vi "Wall Correction.vi"(8 "Direction from car (rad)":dbl[](array[numeric]), 9 "Distance form car":dbl[](array[numeric]), 10 "Y point":dbl[](array[numeric]), 11 "X point":dbl[](array[numeric])) -> (1 "Fix ODM array":dbl[](array[numeric]), 3 "Global Wall Lidar":cluster{dbl[], dbl[]}[](graph))   [LabVIEW 2018]
panel:
  out "VY History 2":T1(graph)
  out "L/R rag":dbl
  out "Up/Down rag":dbl
  out "Wall Distance":dbl[][](array[numeric])
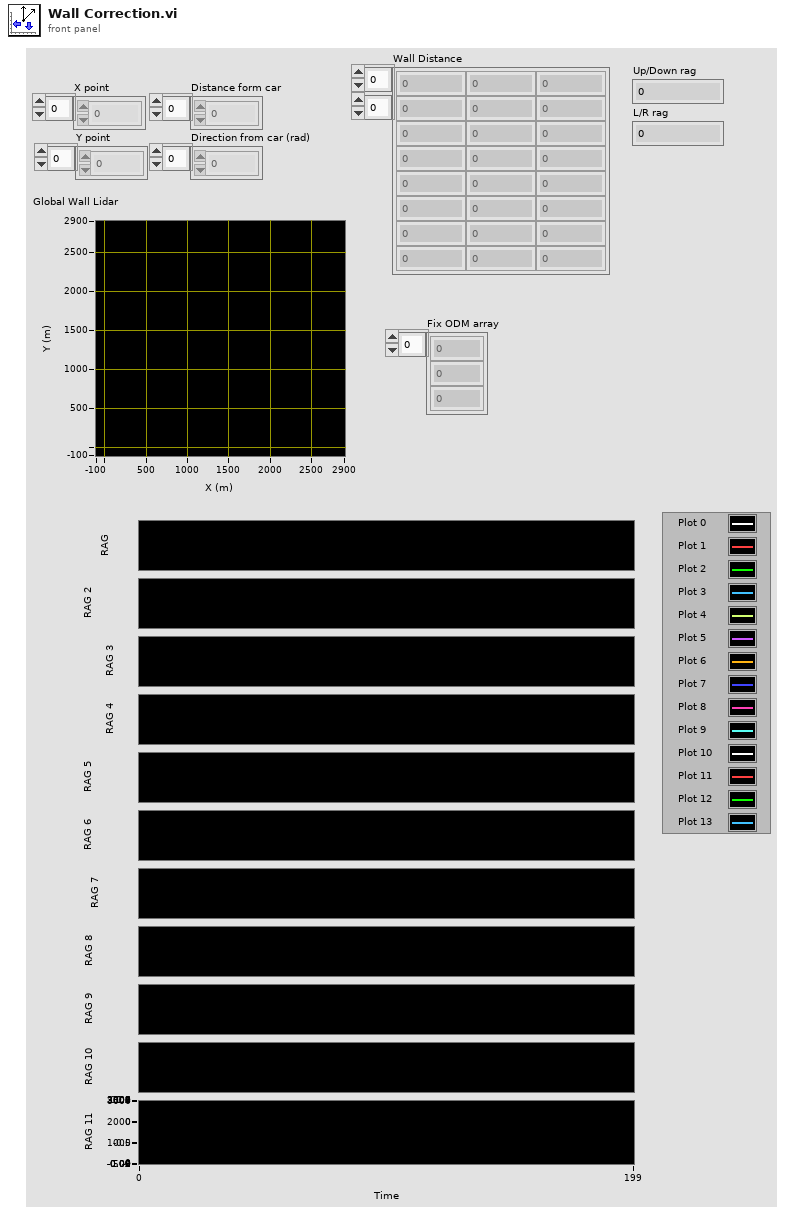
[diagram p1: front panel]
types:
  T1 = cluster{dbl, dbl, "element":dbl, "element":dbl, "element":dbl, "element":dbl, dbl, dbl, dbl, dbl, dbl}
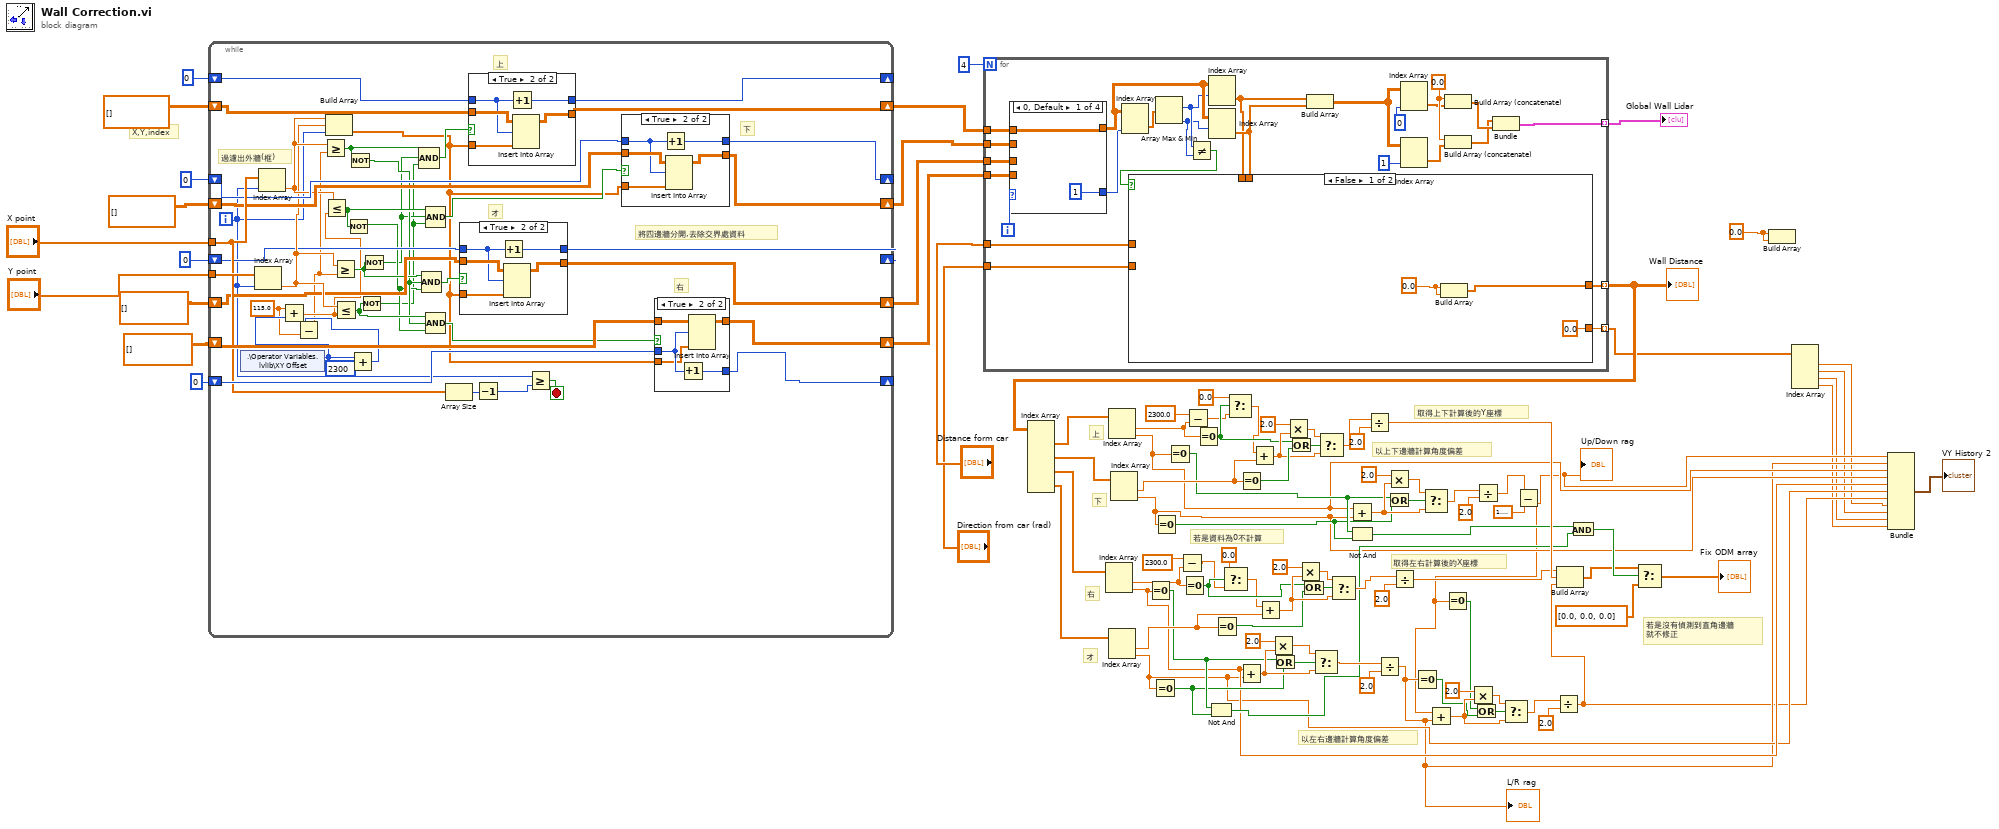
[diagram p0: block diagram]
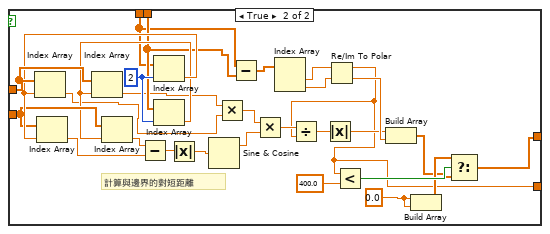
[diagram p2: hidden frame]
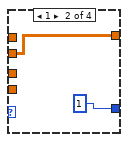
[diagram p3: hidden frame]
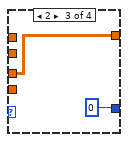
[diagram p4: hidden frame]
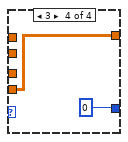
[diagram p5: hidden frame]
diagram:
  w7 = 0.0 ("element")
  # "若是沒有偵測到直角邊牆\n就不修正"
  # "若是資料為0不計算"
  # "以左右邊牆計算角度偏差"
  # "以上下邊牆計算角度偏差"
  # "取得左右計算後的X座標"
  # "取得上下計算後的Y座標"
  # "オ"
  # "右"
  # "下"
  # "上"
  # "X,Y,index"
  n1 = while {
    tunnel: "X point" -> [w138]
    tunnel: "Y point" -> [w142]
    shift-right: [w134] -> w87
    shift-left: dbl[][] [] -> [w141]
    shift-right: [w139] -> _
    shift-left: 0 -> [w140]
    shift-right: [w132] -> _
    shift-left: 0 -> [w133]
    shift-right: [w130] -> w90
    shift-left: dbl[][] [] -> [w131]
    shift-right: [w126] -> _
    shift-left: 0 -> [w129]
    shift-right: [w127] -> w89
    shift-left: dbl[][] [] -> [w128]
    shift-right: [w120] -> _
    shift-left: 0 -> [w123]
    shift-right: [w121] -> w88
    shift-left: dbl[][] [] -> [w122]
    i -> [w112]
    stop <- w135 stop-if-true
    w102 = 115.0 ("lower limit")
    # "右"
    # "オ"
    # "下"
    # "上"
    # "將四邊牆分開,去除交界處資料"
    # "過濾出外牆(框)"
    n2 = shared-variable ".\\Operator Variables.lvlib\\XY Offset"() -> (w104:i16)  [unwired: 1 in, 1 out]
    n3 = Index Array(array=w142, index=w112) -> (element=w124:dbl)
    n4 = Index Array(array=w138, index=w112) -> (element=w125:dbl)
    n5 = Add(x=w102, y=w104) -> (x+y=w105:dbl)
    n6 = Less Or Equal?(x=w125, y=w105) -> (x <= y?=w116:bool)
    n7 = Build Array(w125, w124, w112) -> (w110:dbl[])
    n8 = Less Or Equal?(x=w124, y=w105) -> (x <= y?=w111:bool)
    n9 = Not(x=w116) -> (.not. x?=w108:bool)
    n10 = Add(x=w104, y=i16 2300) -> (x+y=w101:i16)
    n11 = Subtract(x=w101, y=w102) -> (x-y=w100:dbl)
    n12 = Greater Or Equal?(x=w125, y=w100) -> (x >= y?=w117:bool)
    n13 = Greater Or Equal?(x=w124, y=w100) -> (x >= y?=w115:bool)
    n14 = Not(x=w117) -> (.not. x?=w109:bool)
    n15 = Not(x=w111) -> (.not. x?=w106:bool)
    n16 = Not(x=w115) -> (.not. x?=w107:bool)
    n17 = Compound Arithmetic op=AND(w117, w107, w106) -> (w119:bool)
    n18 = Compound Arithmetic op=AND(w115, w109, w108) -> (w114:bool)
    n19 = Compound Arithmetic op=AND(w116, w107, w106) -> (w118:bool)
    n20 = Compound Arithmetic op=AND(w111, w109, w108) -> (w113:bool)
    n21 = Array Size(array=w138) -> (size(s)=w137:i32)
    n22 = case shown="True" w114 {
      tunnel: w123 -> [w151 w152]
      tunnel: [w151 w156] -> w120
      tunnel: w122 -> [w150 w155]
      tunnel: [w150 w154] -> w121
      tunnel: w110 -> [_ w153]
      frame False {
      }
      frame True {
        n23 = Increment(x=w152) -> (x+1=w156:i32)
        n24 = Insert Into Array(array=w155, index (row)=w152, new element=w153) -> (w154:dbl[][])  [unwired: 1 in]
      }
    }
    n25 = case shown="True" w119 {
      tunnel: w133 -> [w165 w166]
      tunnel: [w165 w170] -> w132
      tunnel: w131 -> [w164 w169]
      tunnel: [w164 w168] -> w130
      tunnel: w110 -> [_ w167]
      frame False {
      }
      frame True {
        n26 = Increment(x=w166) -> (x+1=w170:i32)
        n27 = Insert Into Array(array=w169, index (row)=w166, new element=w167) -> (w168:dbl[][])  [unwired: 1 in]
      }
    }
    n28 = Decrement(x=w137) -> (x-1=w136:i32)
    n29 = Greater Or Equal?(x=w112, y=w136) -> (x >= y?=w135:bool)
    n30 = case shown="True" w118 {
      tunnel: w129 -> [w158 w159]
      tunnel: [w158 w163] -> w126
      tunnel: w128 -> [w157 w162]
      tunnel: [w157 w161] -> w127
      tunnel: w110 -> [_ w160]
      frame False {
      }
      frame True {
        n31 = Increment(x=w159) -> (x+1=w163:i32)
        n32 = Insert Into Array(array=w162, index (row)=w159, new element=w160) -> (w161:dbl[][])  [unwired: 1 in]
      }
    }
    n33 = case shown="True" w113 {
      tunnel: w141 -> [w143 w149]
      tunnel: w140 -> [w144 w148]
      tunnel: [w144 w147] -> w139
      tunnel: [w143 w146] -> w134
      tunnel: w110 -> [_ w145]
      frame False {
      }
      frame True {
        n34 = Increment(x=w148) -> (x+1=w147:i32)
        n35 = Insert Into Array(array=w149, index (row)=w148, new element=w145) -> (w146:dbl[][])  [unwired: 1 in]
      }
    }
  }
  n36 = for {
    N: 4 -> [_]
    tunnel: [w187] -> w82 mode=indexing
    tunnel: w90 -> [w185]
    tunnel: w89 -> [w184]
    tunnel: w88 -> [w183]
    tunnel: w87 -> [w182]
    tunnel: "Distance form car" -> [w179]
    tunnel: "Direction from car (rad)" -> [w178]
    tunnel: [w172] -> w28 mode=indexing
    tunnel: [w171] -> w5 mode=indexing
    i -> [w186]
    w194 = 0.0 ("element")
    n37 = case shown="0, Default" w186 {
      tunnel: w185 -> [w230 _ _ _]
      tunnel: w184 -> [_ w232 _ _]
      tunnel: w183 -> [_ _ w234 _]
      tunnel: w182 -> [_ _ _ w236]
      tunnel: [w230 w232 w234 w236] -> w181
      tunnel: [1 ("index") 1 ("index") 0 ("index") 0 ("index")] -> w180
      frame 0, Default {
      }
      frame 1 {
      }
      frame 2 {
      }
      frame 3 {
      }
    }
    n38 = Index Array(array=w181, index (col)=w180) -> (element=w189:dbl[])  [unwired: 1 in]
    n39 = Array Max & Min(array=w189) -> (max index (indices)=w177:i32, min index (indices)=w176:i32)  [unwired: 2 out]
    n40 = Not Equal?(x=w177, y=w176) -> (x != y?=w173:bool)
    n41 = Index Array(array=w181, index (row)=w177) -> (element=w174:dbl[])  [unwired: 1 in]
    n42 = Index Array(array=w181, index (row)=w176) -> (element=w175:dbl[])  [unwired: 1 in]
    n43 = case shown="False" w173 {
      tunnel: w179 -> [_ w224]
      tunnel: w178 -> [_ w222]
      tunnel: w175 -> [_ w217]
      tunnel: w174 -> [_ w216]
      tunnel: [w199 w204] -> w172
      tunnel: [0.0 w200] -> w171
      frame False {
        w198 = 0.0 ("element")
        n44 = Build Array(w198, w198) -> (w199:dbl[])
      }
      frame True {
        w205 = 0.0 ("element")
        w225 = 2 ("index")
        # "計算與邊界的對短距離"
        n45 = Index Array(array=w216, index=w225) -> (element=w223:dbl)
        n46 = Index Array(array=w224, index=w223) -> (element=w213:dbl)
        n47 = Index Array(array=w222, index=w223) -> (element=w219:dbl)
        n48 = Index Array(array=w217, index=w225) -> (element=w221:dbl)
        n49 = Index Array(array=w224, index=w221) -> (element=w214:dbl)
        n50 = Index Array(array=w222, index=w221) -> (element=w220:dbl)
        n51 = Subtract(x=w220, y=w219) -> (x-y=w218:dbl)
        n52 = Absolute Value(x=w218) -> (abs(x)=w215:dbl)
        n53 = Sine & Cosine(0:w215) -> (1:w211:dbl)  [unwired: 1 out]
        n54 = Multiply(x=w214, y=w213) -> (x*y=w212:dbl)
        n55 = Subtract(x=w216, y=w217) -> (x-y=w226:dbl[])
        n56 = Multiply(x=w212, y=w211) -> (x*y=w210:dbl)
        n57 = Index Array(array=w226) -> (element #1=w227:dbl, element #2=w228:dbl)  [unwired: 2 in]
        n58 = Re/Im To Polar(2:w228, 3:w227) -> (0:w209:dbl, 1:w200:dbl)
        n59 = Divide(x=w210, y=w200) -> (x/y=w208:dbl)
        n60 = Absolute Value(x=w208) -> (abs(x)=w207:dbl)
        n61 = Less?(x=w200, y=400.0) -> (x < y?=w203:bool)
        n62 = Build Array(w207, w209) -> (w201:dbl[])
        n63 = Build Array(w205, w205) -> (w202:dbl[])
        n64 = Select(t=w202, s=w203, f=w201) -> (s? t:f=w204:dbl[])
      }
    }
    n65 = Build Array(w174, w175) -> (w188:dbl[][])
    n66 = Index Array(array=w188, index (col)=0 ("disabled index (col)")) -> (element=w191:dbl[])  [unwired: 1 in]
    n67 = Index Array(array=w188, index (col)=1 ("disabled index (col)")) -> (element=w190:dbl[])  [unwired: 1 in]
    n68 = Build Array (concatenate)(w194, w191) -> (w196:dbl[])
    n69 = Build Array (concatenate)(w194, w190) -> (w195:dbl[])
    n70 = Bundle(w195, w196) -> (w187:cluster{dbl[], dbl[]})  [unwired: 1 in]
  }
  "Global Wall Lidar" <- w82
  "Wall Distance" <- w28
  n71 = Index Array(array=w28) -> (element #1=w81:dbl[], element #2=w29:dbl[], element #3=w80:dbl[], element #4=w79:dbl[])  [unwired: 8 in]
  n72 = Index Array(array=w80) -> (element #1=w75:dbl, element #2=w11:dbl)  [unwired: 2 in]
  n73 = Index Array(array=w79) -> (element #1=w64:dbl, element #2=w10:dbl)  [unwired: 2 in]
  n74 = Index Array(array=w81) -> (element #1=w76:dbl, element #2=w13:dbl)  [unwired: 2 in]
  n75 = Index Array(array=w29) -> (element #1=w74:dbl, element #2=w12:dbl)  [unwired: 2 in]
  n76 = Equal To 0?(x=w11) -> (x = 0?=w19:bool)
  n77 = Equal To 0?(x=w10) -> (x = 0?=w18:bool)
  n78 = Equal To 0?(x=w12) -> (x = 0?=w20:bool)
  n79 = Equal To 0?(x=w13) -> (x = 0?=w21:bool)
  n80 = Subtract(x=2300.0, y=w75) -> (x-y=w34:dbl)
  n81 = Equal To 0?(x=w75) -> (x = 0?=w35:bool)
  n82 = Subtract(x=2300.0, y=w76) -> (x-y=w38:dbl)
  n83 = Equal To 0?(x=w76) -> (x = 0?=w39:bool)
  n84 = Not And(1:w18, 2:w19) -> (0:w17:bool)
  n85 = Equal To 0?(x=w64) -> (x = 0?=w30:bool)
  n86 = Select(t=0.0, s=w35, f=w34) -> (s? t:f=w32:dbl)
  n87 = Select(t=0.0, s=w39, f=w38) -> (s? t:f=w36:dbl)
  n88 = Equal To 0?(x=w74) -> (x = 0?=w72:bool)
  n89 = Add(x=w11, y=w10) -> (x+y=w58:dbl)
  n90 = Add(x=w36, y=w74) -> (x+y=w69:dbl)
  n91 = Add(x=w32, y=w64) -> (x+y=w68:dbl)
  n92 = Multiply(x=2.0, y=w58) -> (x*y=w60:dbl)
  n93 = Or(x=w19, y=w18) -> (x .or. y?=w26:bool)
  n94 = Multiply(x=2.0, y=w69) -> (x*y=w71:dbl)
  n95 = Or(x=w39, y=w72) -> (x .or. y?=w73:bool)
  n96 = Multiply(x=2.0, y=w68) -> (x*y=w66:dbl)
  n97 = Or(x=w35, y=w30) -> (x .or. y?=w65:bool)
  n98 = Select(t=w60, s=w26, f=w58) -> (s? t:f=w50:dbl)
  n99 = Select(t=w71, s=w73, f=w69) -> (s? t:f=w57:dbl)
  n100 = Select(t=w66, s=w65, f=w68) -> (s? t:f=w51:dbl)
  n101 = Add(x=w13, y=w12) -> (x+y=w63:dbl)
  n102 = Not And(1:w20, 2:w21) -> (0:w16:bool)
  n103 = Divide(x=w57, y=2.0 ("x")) -> (x/y=w48:dbl)
  n104 = Divide(x=w50, y=2.0 ("x")) -> (x/y=w9:dbl)
  "L/R rag" <- w9
  n105 = Multiply(x=2.0, y=w63) -> (x*y=w61:dbl)
  n106 = Or(x=w21, y=w20) -> (x .or. y?=w27:bool)
  n107 = Divide(x=w51, y=2.0 ("x")) -> (x/y=w31:dbl)
  n108 = Equal To 0?(x=w9) -> (x = 0?=w40:bool)
  n109 = Select(t=w61, s=w27, f=w63) -> (s? t:f=w55:dbl)
  n110 = Divide(x=w55, y=2.0 ("x")) -> (x/y=w15:dbl)
  n111 = Subtract(x=w15, y=1.5707963267948966) -> (x-y=w6:dbl)
  "Up/Down rag" <- w6
  n112 = Add(x=w6, y=w9) -> (x+y=w42:dbl)
  n113 = Equal To 0?(x=w6) -> (x = 0?=w41:bool)
  n114 = Multiply(x=2.0, y=w42) -> (x*y=w44:dbl)
  n115 = Or(x=w41, y=w40) -> (x .or. y?=w45:bool)
  n116 = Select(t=w44, s=w45, f=w42) -> (s? t:f=w46:dbl)
  n117 = Divide(x=w46, y=2.0 ("x")) -> (x/y=w8:dbl)
  n118 = Build Array(w31, w48, w8) -> (w24:dbl[])
  n119 = And(x=w16, y=w17) -> (x .and. y?=w25:bool)
  n120 = Select(t=w24, s=w25, f=dbl[] [0.0, 0.0, 0.0] ("Fix ODM array")) -> (s? t:f=→"Fix ODM array":dbl[])
  n121 = Build Array(w7, w7) -> ()  [unwired: 1 out]
  n122 = Index Array(array=w5) -> (element #1=w4:dbl, element #2=w3:dbl, element #3=w2:dbl, element #4=w1:dbl)  [unwired: 4 in]
  n123 = Bundle(w6, w9, "element"=w13, "element"=w12, "element"=w11, "element"=w10, w8, w4, w3, w2, w1) -> (→"VY History 2":T1)  [unwired: 1 in]
